vi "Read Numeric Wrapper.vi"(8 "error in (no error)":errorcluster, 11 "ModifiedClass in":refnum<class "ModifiedClass.lvclass">) -> (0 "error out":errorcluster, 1 "LV Class Version":string, 2 "Numeric":dbl, 3 "ModifiedClass out":refnum<class "ModifiedClass.lvclass">)   [LabVIEW 2009]
uses:
  ModifiedClass.lvclass
panel:
  in  "LV Class File Path":string="ModifiedClass.lvclass"
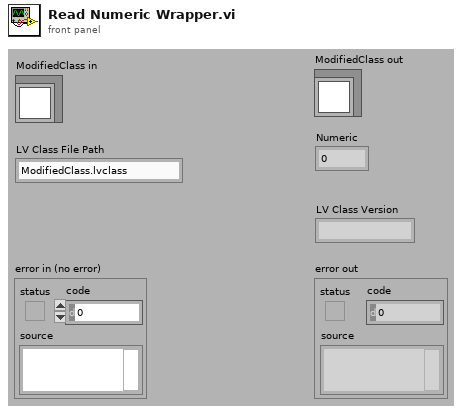
[diagram p1: front panel]
types:
  T1 = cluster{"Major":u16, "Minor":u16, "Fix":u16, "Build":u16}
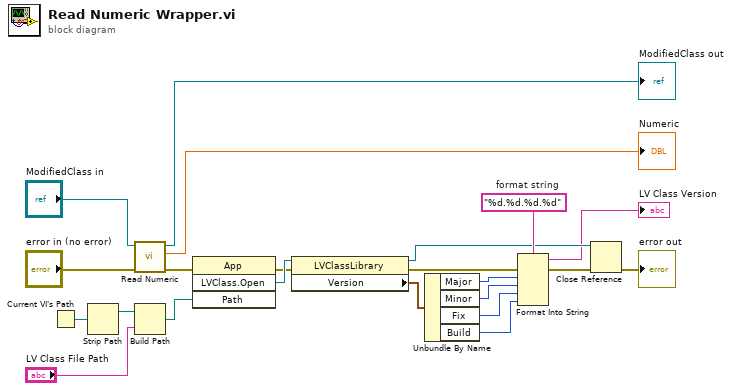
[diagram p0: block diagram]
diagram:
  w7 = "%d.%d.%d.%d"  # format string
  n1 = Current VI's Path() -> (path=w18:path)
  n2 = Strip Path(path=w18) -> (stripped path=w17:path)  [unwired: 1 out]
  n3 = call-dynamic "Read Numeric.vi"("error in (no error)"="error in (no error)", "ModifiedClass in"="ModifiedClass in") -> ("error out"=w14:errorcluster, "Numeric"=→"Numeric":dbl, "ModifiedClass out"=→"ModifiedClass out":refnum<class "ModifiedClass.lvclass">)  [unwired: 7 in]
  n4 = Build Path(base path=w17, name or relative path="LV Class File Path") -> (appended path=w15:path)
  n5 = invoke class="App" method="LVClass.Open"(error in=w14, "Path"=w15) -> (error out=w12:errorcluster, "LVClass.Open"=w13:refnum<vi>)  [unwired: 2 in, 2 out]
  n6 = property class="LVClassLibrary"(reference=w13, error in=w12) -> (reference out=w5:refnum<vi>, error out=w4:errorcluster, "Version"=w3:T1)
  n7 = Unbundle By Name(w3) -> ("Major"=w11:u16, "Minor"=w10:u16, "Fix"=w9:u16, "Build"=w8:u16)
  n8 = Format Into String(format string=w7, error in=w4, w11, w10, w9, w8) -> (resulting string=→"LV Class Version":string, error out=w6:errorcluster)  [unwired: 1 in]
  n9 = Close Reference(reference=w5, error in (no error)=w6) -> (error out=→"error out":errorcluster)
